vi "ImPro - Reset Visible.vi"(8 "error in (no error)":errorcluster, 11 "output cluster":T1) -> (0 "error out":errorcluster)   [LabVIEW 2023]
uses:
  Controls/ImPro - UI Refs.ctl
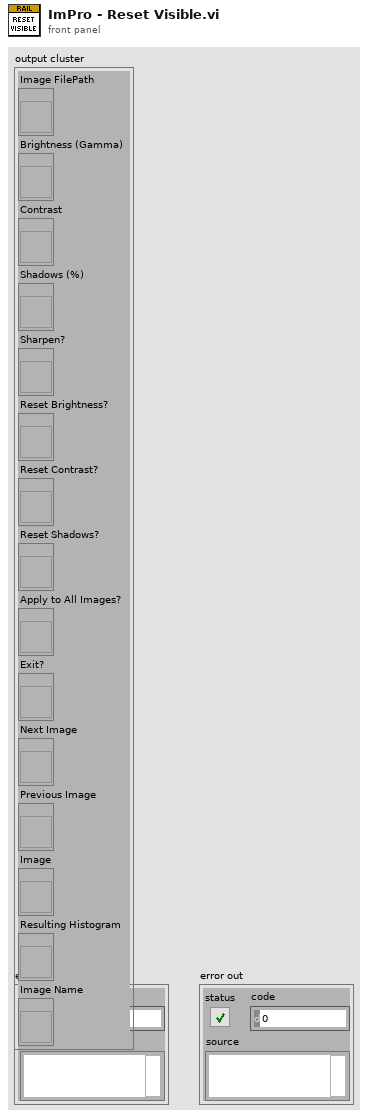
[diagram p1: front panel]
types:
  T1 = typedef "ImPro - UI Refs.ctl" = cluster{"Image FilePath":refnum<vi>, "Brightness (Gamma)":refnum<vi>, "Contrast":refnum<vi>, "Shadows (%)":refnum<vi>, "Sharpen?":refnum<vi>, "Reset Brightness?":refnum<vi>, "Reset Contrast?":refnum<vi>, "Reset Shadows?":refnum<vi>, "Apply to All Images?":refnum<vi>, "Exit?":refnum<vi>, "Next Image":refnum<vi>, "Previous Image":refnum<vi>, "Image":refnum<vi>, "Resulting Histogram":refnum<vi>, "Image Name":refnum<vi>}
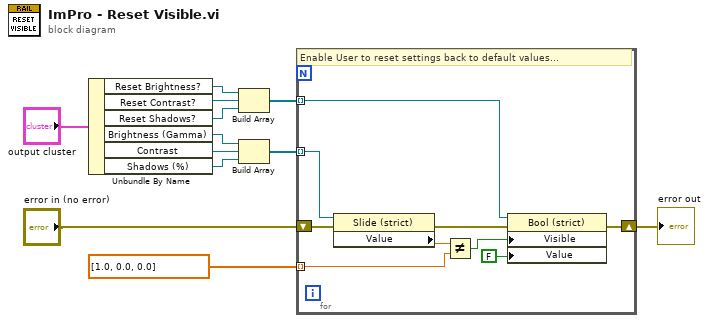
[diagram p0: block diagram]
diagram:
  n1 = Unbundle By Name("output cluster") -> ("Reset Brightness?"=w7:refnum<vi>, "Reset Contrast?"=w6:refnum<vi>, "Reset Shadows?"=w5:refnum<vi>, "Brightness (Gamma)"=w4:refnum<vi>, "Contrast"=w3:refnum<vi>, "Shadows (%)"=w2:refnum<vi>)
  n2 = Build Array(w7, w6, w5) -> (w12:refnum<vi>[])
  n3 = Build Array(w4, w3, w2) -> (w11:refnum<vi>[])
  n4 = for {
    shift-right: [w15] -> w9
    shift-left: "error in (no error)" -> [w21]
    tunnel: w11 -> [w20] mode=indexing
    tunnel: w12 -> [w16] mode=indexing
    tunnel: dbl[] [1.0, 0.0, 0.0] -> [w18] mode=indexing
    # "Enable User to reset settings back to default values..."
    n5 = property class="Slide (strict)"(reference=w20, error in=w21) -> (error out=w17:errorcluster, "Value"=w19:dbl)  [unwired: 1 out]
    n6 = Not Equal?(x=w19, y=w18) -> (x != y?=w14:bool)
    n7 = property class="Bool (strict)"(reference=w16, error in=w17, "Visible"=w14, "Value"=FALSE) -> (error out=w15:errorcluster)  [unwired: 1 out]
  }
  "error out" <- w9
